vi "Save File Comments.vi"(8 "error in (no error)":errorcluster, 9 "filename struct":T1, 10 "base file name":string="test", 11 "folder path":path=path "C:/") -> (0 "error out":errorcluster, 2 "test discarded?":bool, 3 "controller data":T2)   [LabVIEW 2020]
uses:
  Controller Loop/Message and Data.ctl
  Inflation Test/Parameter Class/IA Test Parameters.lvclass
  Controllers/Controller.lvclass
  Hardware/Sensors/Cameras/Camera.lvclass
  Hardware/Sensors/Force Sensors/Force Sensor.lvclass
  Hardware/Actuators/Servos/Servo.lvclass
  Hardware/Actuators/Switches/Switch.lvclass
  Filename Structure.ctl
panel:
  in  "discard test":bool
  in  "save test":bool
  in  "comments":string="Aorta Type: <>, Inner Diameter: <XX.X>mm, Outer Diameter: <XX.X>mm, Initial Wall Thickness: <X.XX>mm, Aorta Location: <>"
  # "TEST COMMENTS"
  # "DO YOU WANT TO SAVE ANY COMMENTS TO THE FILE REGARDING THE TEST?"
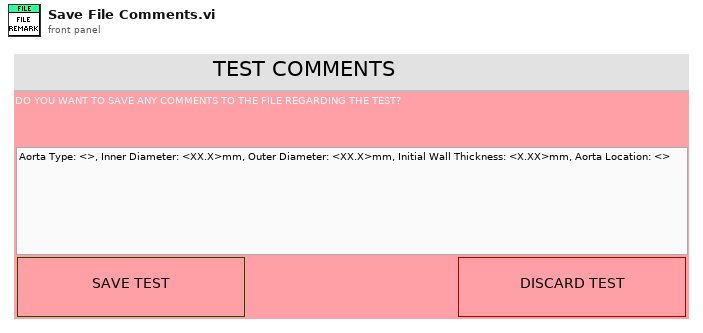
[diagram p1: front panel]
types:
  T1 = typedef "Filename Structure.ctl" = enum16{"<nameYYYYMMDDi>", "<name>"}
  T2 = typedef "Message and Data.ctl" = cluster{"msg":string, "ia test param":refnum<class "IA Test Parameters.lvclass">, "controller type":refnum<class "Controller.lvclass">, "folder path":path, "file name":string, "file comments":string, "cam":refnum<class "Camera.lvclass">, "fs":refnum<class "Force Sensor.lvclass">, "servo":refnum<class "Servo.lvclass">, "switch":refnum<class "Switch.lvclass">, "filename struct":T1}
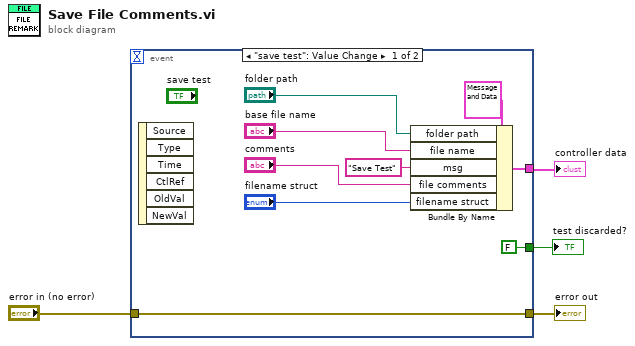
[diagram p0: block diagram]
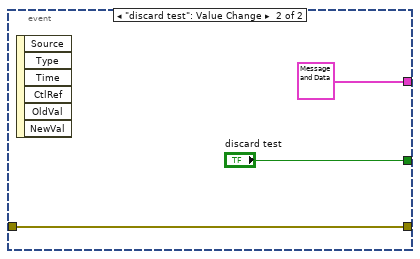
[diagram p2: hidden frame]
diagram:
  n1 = event shown="[0] \"save test\": Value Change" {
    selector: _ -> [_ _]
    dyn-events: _ -> [_ _]
    timeout: _ -> [_ _]
    tunnel: [w13 w15] -> w4
    tunnel: "error in (no error)" -> [w13 w15]
    tunnel: [w6 T2 {"msg"="", "ia test param"=refnum, "controller type"=refnum, "folder path"=path "", "file name"="", "file comments"="", "cam"=refnum, "fs"=refnum, "servo"=refnum, "switch"=refnum, "filename struct"=enum."<nameYYYYMMDDi>"} ("element")] -> w2
    tunnel: [FALSE ("discard test") "discard test"] -> w1
    event "save test": Value Change {
      n2 = event-data() -> ()  [unwired: 1 in, 6 out]
      n3 = Bundle By Name(cluster=T2 {"msg"="", "ia test param"=refnum, "controller type"=refnum, "folder path"=path "", "file name"="", "file comments"="", "cam"=refnum, "fs"=refnum, "servo"=refnum, "switch"=refnum, "filename struct"=enum."<nameYYYYMMDDi>"} ("element"), "folder path"="folder path", "file name"="base file name", "msg"="Save Test", "file comments"="comments", "filename struct"="filename struct") -> (w6:T2)
    }
    event "discard test": Value Change {
      n4 = event-data() -> ()  [unwired: 1 in, 6 out]
    }
  }
  "controller data" <- w2
  "error out" <- w4
  "test discarded?" <- w1
